vi "niRFUtil WFM Compensate IQ Gain Imbalance.vi"(0 "Input":T1 {"y" format="%.2f"; "dx" format="%^.2e"; "x0" format="%^.2e"}, 2 "Gain Imablance (lin)":dbl, 3 "Compensate?":bool) -> (7 "Waveform Out":T1 {"y" format="%.2f"; "dx" format="%^.2e"; "x0" format="%^.2e"})   [LabVIEW 2015, in "niRFUtil.lvlib"]
uses:
  niRFUtil.lvlib
  Includes/niRFUtil INC Complex Waveform.ctl
  Includes/niRFUtil INC Complex Array.ctl
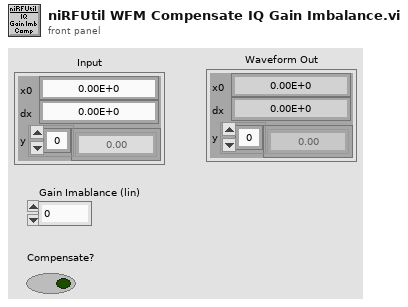
[diagram p1: front panel]
types:
  T1 = typedef "niRFUtil.lvlib/niRFUtil INC Complex Waveform.ctl" = cluster{"x0":dbl, "dx":dbl, "y":T2}
  T2 = typedef "niRFUtil.lvlib/niRFUtil INC Complex Array.ctl" = csg[]
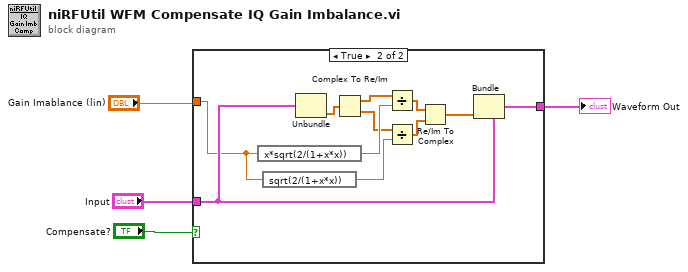
[diagram p0: block diagram]
diagram:
  n1 = case shown="True" "Compensate?" {
    tunnel: "Input" -> [w5 w13]
    tunnel: [w5 w14] -> w4
    tunnel: "Gain Imablance (lin)" -> [_ w6]
    frame False {
    }
    frame True {
      n2 = expression code="x*sqrt(2/(1+x*x))"(w6) -> (w11:dbl)
      n3 = expression code="sqrt(2/(1+x*x))"(w6) -> (w9:dbl)
      n4 = Unbundle(w13) -> ("y"=w15:T2)  [unwired: 2 out]
      n5 = Complex To Re/Im(x + iy=w15) -> (x=w12:sgl[], y=w10:sgl[])
      n6 = Divide(x=w12, y=w11) -> (x/y=w7:dbl[])
      n7 = Divide(x=w10, y=w9) -> (x/y=w8:dbl[])
      n8 = Re/Im To Complex(1:w8, 2:w7) -> (0:w16:cdb[])
      n9 = Bundle(cluster=w13, "y"=w16) -> (w14:T1)  [unwired: 2 in]
    }
  }
  "Waveform Out" <- w4
